vi "CAN_Heartbeat_switch.vi"(8 "error in":errorcluster, 11 "CAN_Hearbeat_boolVar":bool) -> (0 "error out":errorcluster)   [LabVIEW 2009, in "OWNCAN.lvlib"]
uses:
  OWNCAN.lvlib
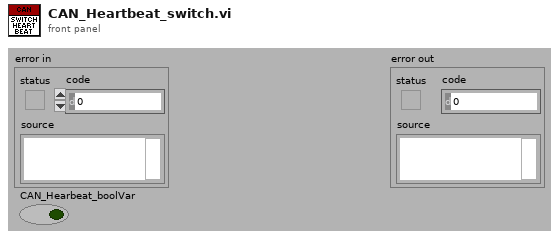
[diagram p1: front panel]
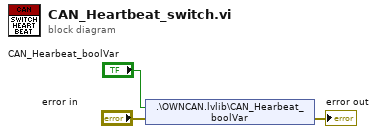
[diagram p0: block diagram]
diagram:
  n1 = shared-variable ".\\OWNCAN.lvlib\\CAN_Hearbeat_boolVar"("CAN_Hearbeat_boolVar", error in="error in") -> (error out=→"error out":errorcluster)
